vi "Parse CD Notifier Data V2.vi"(9 "Status Hdr Length":i32, 10 "Pixel Array Length":u32, 11 "Sample Data Array":u32[](array[numeric])) -> (0 "Last Sample":u32[](array[numeric]), 1 "Encoder Out":i32, 2 "nSamples":u32, 3 "Last Sample No.":u32, 4 "Array Header":u32[](array[numeric]))   [LabVIEW 2015, in "Collect Data Mgr.lvlib"]
uses:
  Collect Data Mgr.lvlib
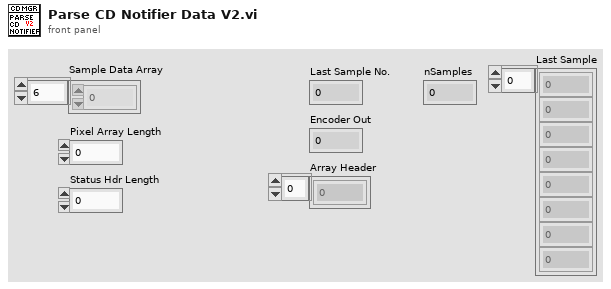
[diagram p1: front panel]
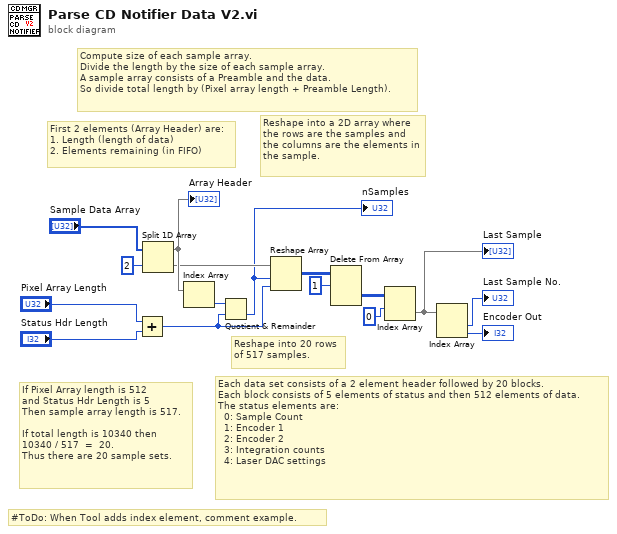
[diagram p0: block diagram]
diagram:
  # "#ToDo: When Tool adds index element, comment example."
  # "Reshape into 20 rows of 517 samples."
  # "Reshape into a 2D array where the rows are the samples and the columns are the elements in the sample."
  # "Compute size of each sample array.\nDivide the length by the size of each sample array.\nA sample array consists of a Preamble and the data.\nSo divide total length by (Pixel array length + Preamble Length)."
  # "First 2 elements (Array Header) are:\n1. Length (length of data)\n2. Elements remaining (in FIFO)"
  # "If Pixel Array length is 512\nand Status Hdr Length is 5\nThen sample array length is 517.\n\nIf total length is 10340 then \n10340 / 517  =  20.\nThus there are 20 sample sets."
  # "Each data set consists of a 2 element header followed by 20 blocks.\nEach block consists of 5 elements of status and then 512 elements of data.\nThe status elements are:\n  0: Sample Count\n  1: Encoder 1\n  2: Encoder 2\n  3: Integration counts\n  4: Laser DAC settings"
  n1 = Add(x="Pixel Array Length", y="Status Hdr Length") -> (x+y=w8:u32)
  n2 = Split 1D Array(array="Sample Data Array", index=2) -> (first subarray=w11:u32[], second subarray=w10:u32[])
  "Array Header" <- w11
  n3 = Index Array(array=w11) -> (element=w12:u32)  [unwired: 1 in]
  n4 = Quotient & Remainder(x=w12, y=w8) -> (floor(x/y)=w9:u32)  [unwired: 1 out]
  "nSamples" <- w9
  n5 = Reshape Array(w10, w9, w8) -> (w7:u32[][])
  n6 = Delete From Array(array=w7, length=1) -> (deleted portion=w5:u32[][])  [unwired: 2 in, 1 out]
  n7 = Index Array(array=w5, index (row)=0 ("disabled index (col)")) -> (element=w3:u32[])  [unwired: 1 in]
  "Last Sample" <- w3
  n8 = Index Array(array=w3) -> (element #1=→"Last Sample No.":u32, element #2=→"Encoder Out":u32)  [unwired: 2 in]
